vi "Init Bfr Rx - Create Channels.vi"(5 "External Buffer":bool, 7 "Packet Name":string, 8 "error in (no error)":errorcluster, 10 "Rx Buffer Option":T1, 11 "Data Access":refnum<class "Data Access Engine.lvclass">) -> (0 "error out":errorcluster, 3 "Buffered Receive Channels":T2)   [LabVIEW 2019, in "UDP-Custom-Device Engine.lvlib"]
uses:
  UDP-Custom-Device Engine.lvlib
  Types/Engine - Buffered Rx Channel Refs.ctl
  <vilib>/NI/NIVS Inline Async API/_Data Access Engine/Data Access Engine/Types/Write.DVR.ctl
  <vilib>/NI/NIVS Inline Async API/_Data Access Engine/Access Type Classes/Write/Write.lvclass
  <vilib>/NI/NIVS Inline Async API/_Data Access Engine/Data Access Engine/Types/Read.DVR.ctl
  <vilib>/NI/NIVS Inline Async API/_Data Access Engine/Access Type Classes/Read/Read.lvclass
  Types/Engine - Buffered Rx Ping Pong Channels.ctl
  <vilib>/NI/NIVS Inline Async API/_Data Access Engine/Data Access Engine/Data Access Engine.lvclass
  Shared/Types/Shared - Receive Buffer Options.ctl
  <vilib>/NI/NIVS Inline Async API/_Data Access Engine/Data Access Engine/Methods/Write.Lookup.vi
  <vilib>/NI/NIVS Inline Async API/_Data Access Engine/Data Access Engine/Methods/Read.Lookup.vi
  Shared/UDP-Custom-Device Shared.lvlib
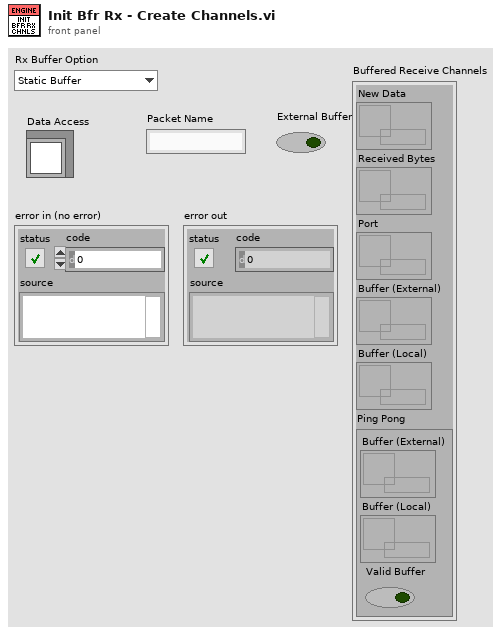
[diagram p1: front panel]
types:
  T1 = typedef "UDP-Custom-Device Shared.lvlib/Shared - Receive Buffer Options.ctl" = enum16{"Static Buffer", "Circular Buffer", "Circular Buffer + Size", "Internal Cache", "Internal Cache + Size", "Ping Pong", "Ping Pong + Size"}
  T2 = typedef "UDP-Custom-Device Engine.lvlib/Engine - Buffered Rx Channel Refs.ctl" = cluster{"New Data":T3, "Received Bytes":T3, "Port":T3, "Buffer (External)":T4, "Buffer (Local)":T3, "Ping Pong":T5}
  T3 = typedef "Data Access Engine.lvlib/Data Access Engine.lvclass/Write.DVR.ctl" = refnum<data-value>
  T4 = typedef "Data Access Engine.lvlib/Data Access Engine.lvclass/Read.DVR.ctl" = refnum<data-value>
  T5 = typedef "UDP-Custom-Device Engine.lvlib/Engine - Buffered Rx Ping Pong Channels.ctl" = cluster{"Buffer (External)":T4, "Buffer (Local)":T3, "Valid Buffer":bool}
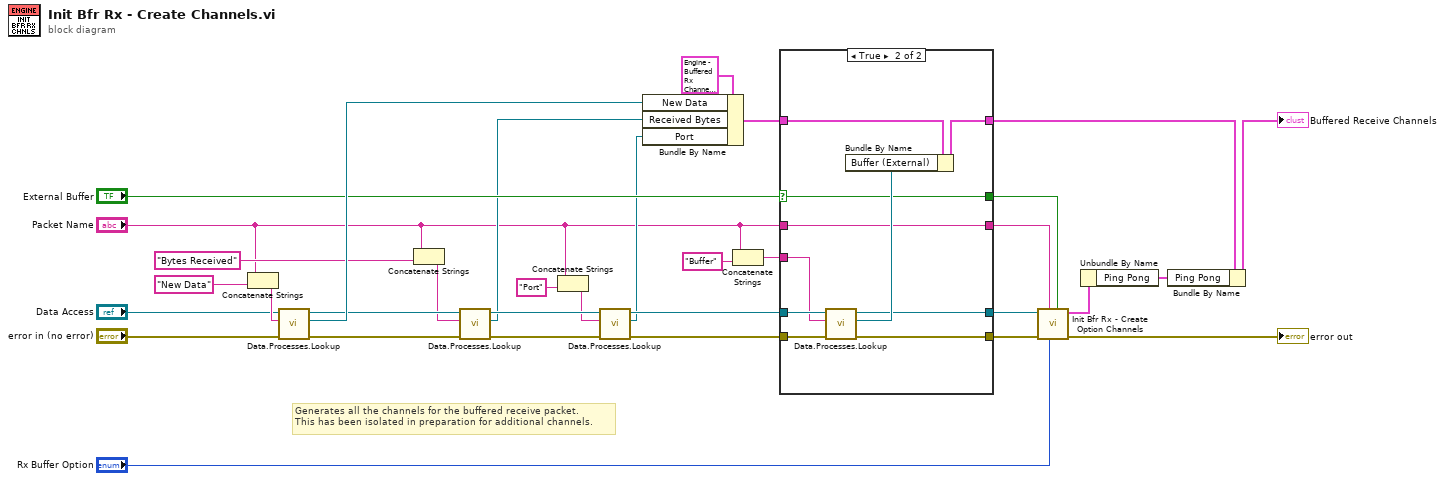
[diagram p0: block diagram]
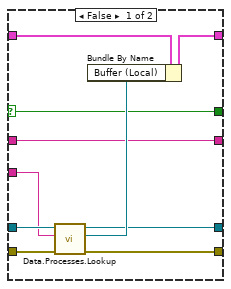
[diagram p2: hidden frame]
diagram:
  # "Generates all the channels for the buffered receive packet.\nThis has been isolated in preparation for additional channels."
  n1 = Concatenate Strings("Packet Name", "New Data" ("Item GUID")) -> (w33:string)
  n2 = call-poly <vilib>:"Data.Processes.Lookup.vi"("error in (no error)"="error in (no error)", "Name"=w33, "Data Access API in"="Data Access") -> ("error out"=w25:errorcluster, "Ref"=w28:T3, "Data Access API out"=w19:refnum<class "Data Access Engine.lvclass">)  [unwired: 5 in, 1 out]
  n3 = Concatenate Strings("Packet Name", "Bytes Received" ("string")) -> (w13:string)
  n4 = call-poly <vilib>:"Data.Processes.Lookup.vi"("error in (no error)"=w25, "Name"=w13, "Data Access API in"=w19) -> ("error out"=w24:errorcluster, "Ref"=w12:T3, "Data Access API out"=w18:refnum<class "Data Access Engine.lvclass">)  [unwired: 5 in, 1 out]
  n5 = Concatenate Strings("Packet Name", "Port" ("Item GUID")) -> (w15:string)
  n6 = call-poly <vilib>:"Data.Processes.Lookup.vi"("error in (no error)"=w24, "Name"=w15, "Data Access API in"=w18) -> ("error out"=w23:errorcluster, "Ref"=w14:T3, "Data Access API out"=w17:refnum<class "Data Access Engine.lvclass">)  [unwired: 5 in, 1 out]
  n7 = Bundle By Name(cluster=T2 {"New Data"=refnum, "Received Bytes"=refnum, "Port"=refnum, "Buffer (External)"=refnum, "Buffer (Local)"=refnum, "Ping Pong"={"Buffer (External)"=refnum, "Buffer (Local)"=refnum, "Valid Buffer"=FALSE}} ("Buffered Receive Channels"), "New Data"=w28, "Received Bytes"=w12, "Port"=w14) -> (w26:T2)
  n8 = Concatenate Strings("Packet Name", "Buffer" ("Item GUID")) -> (w16:string)
  n9 = case shown="True" "External Buffer" {
    selector: "External Buffer" -> [w36 w46]
    tunnel: [w39 w49] -> w3
    tunnel: w26 -> [w40 w50]
    tunnel: [w37 w47] -> w10
    tunnel: w23 -> [w38 w48]
    tunnel: w17 -> [w43 w53]
    tunnel: w16 -> [w42 w52]
    tunnel: [w36 w46] -> w8
    tunnel: [w35 w45] -> w7
    tunnel: "Packet Name" -> [w35 w45]
    tunnel: [w34 w44] -> w5
    frame False {
      n10 = call-poly <vilib>:"Data.Processes.Lookup.vi"("error in (no error)"=w38, "Name"=w42, "Data Access API in"=w43) -> ("error out"=w37:errorcluster, "Ref"=w41:T3, "Data Access API out"=w34:refnum<class "Data Access Engine.lvclass">)  [unwired: 5 in, 1 out]
      n11 = Bundle By Name(cluster=w40, "Buffer (Local)"=w41) -> (w39:T2)
    }
    frame True {
      n12 = call-poly <vilib>:"Data.Processes.Lookup.vi"("error in (no error)"=w48, "Name"=w52, "Data Access API in"=w53) -> ("error out"=w47:errorcluster, "Ref"=w51:T4, "Data Access API out"=w44:refnum<class "Data Access Engine.lvclass">)  [unwired: 5 in, 1 out]
      n13 = Bundle By Name(cluster=w50, "Buffer (External)"=w51) -> (w49:T2)
    }
  }
  n14 = call "Init Bfr Rx - Create Option Channels.vi"("External Buffer"=w8, "Rx Buffer Option"="Rx Buffer Option", "Packet Name"=w7, "error in (no error)"=w10, "Data Access"=w5) -> ("error out"=→"error out":errorcluster, "Buffer Options"=w2:cluster{"Ping Pong":T5})  [unwired: 5 in]
  n15 = Unbundle By Name(w2) -> ("Ping Pong"=w1:T5)
  n16 = Bundle By Name(cluster=w3, "Ping Pong"=w1) -> (→"Buffered Receive Channels":T2)
